vi "Do.vi"(8 "error in (no error)":errorcluster, 10 "Actor in":refnum<class "Actor.lvclass">, 11 "Preview Stack Msg":refnum<class "Preview Stack Msg.lvclass">) -> (0 "error out":errorcluster, 2 "Actor out":refnum<class "Actor.lvclass">)   [LabVIEW 2012, in "UPNCalculator Actor.lvlib" / "Preview Stack Msg.lvclass"]
doc: "This VI delivers the message to the actor by calling the appropriate method(s) on the actor."
uses:
  Preview Stack Msg.lvclass
  <vilib>/ActorFramework/Actor/Actor.lvclass
  UPNCalculator/UPNCalculator.lvclass
  Preview Stack Msg.lvclass/Preview Stack Msg.ctl
  Calculator/Calculator Messages/Display Result Msg/Display Result Msg.lvclass/Display Result Msg.ctl
  <vilib>/ActorFramework/Message Enqueuer/Message Enqueuer.lvclass/Message Enqueuer.ctl
  <vilib>/ActorFramework/Message Enqueuer/Enqueue.vi
  <vilib>/ActorFramework/Message Priority Queue/Priority Enqueue.vi
  Calculator/Calculator Messages/Display Result Msg/Display Result Msg.lvclass
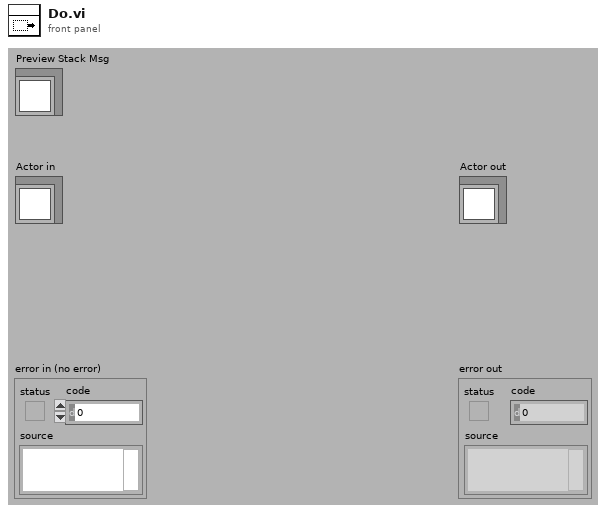
[diagram p1: front panel]
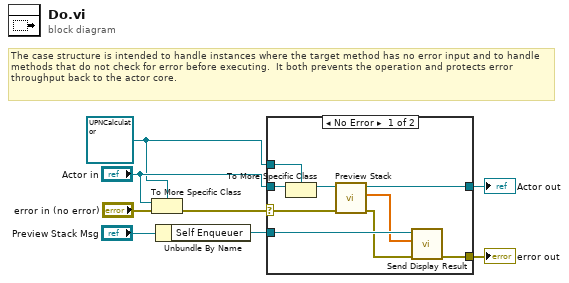
[diagram p0: block diagram]
diagram:
  w3 = refnum<class "UPNCalculator.lvclass"> refnum ("Actor in")
  # "The case structure is intended to handle instances where the target method has no error input and to handle methods that do not check for error before executing.  It both prevents the operation and protects error throughput back to the actor core."
  n1 = To More Specific Class(target class=w3, reference="Actor in", error in="error in (no error)") -> (error out=w7:errorcluster)  [unwired: 1 out]
  n2 = Unbundle By Name("Preview Stack Msg") -> ("Self Enqueuer"=w1:refnum<class "Message Enqueuer.lvclass">)
  n3 = case shown="No Error" w7 {
    selector: w7 -> [w16 w19]
    tunnel: [w9 w19] -> w6
    tunnel: [w17 w18] -> w5
    tunnel: "Actor in" -> [w15 w18]
    tunnel: w3 -> [w14 _]
    tunnel: w1 -> [w12 _]
    frame No Error {
      n4 = To More Specific Class(target class=w14, reference=w15) -> (specific class reference=w13:refnum<class "UPNCalculator.lvclass">)  [unwired: 1 in, 1 out]
      n5 = call "Preview Stack.vi"("error in (no error)"=w16, "UPNCalculator in"=w13) -> ("error out"=w10:errorcluster, "Stack"=w11:dbl[], "UPNCalculator out"=w17:refnum<class "UPNCalculator.lvclass">)  [unwired: 7 in]
      n6 = call "Send Display Result.vi"("error in (no error)"=w10, "Stack"=w11, "Message Enqueuer"=w12) -> ("error out"=w9:errorcluster)  [unwired: 7 in, 1 out]
    }
    frame Error {
      # "If type check fails, pass the original object out again."
    }
  }
  "error out" <- w6
  "Actor out" <- w5
